vi "Write FFT Window.vi"(8 "error in (no error)":errorcluster, 10 "FFT Window":dbl, 11 "MOCKBEAR in":refnum<class "MOCKBEAR.lvclass">) -> (0 "error out":errorcluster, 3 "MOCKBEAR out":refnum<class "MOCKBEAR.lvclass">)   [LabVIEW 2021, in "MOCKBEAR.lvclass"]
uses:
  MOCKBEAR.lvclass
  MOCKBEAR.lvclass/MOCKBEAR.ctl
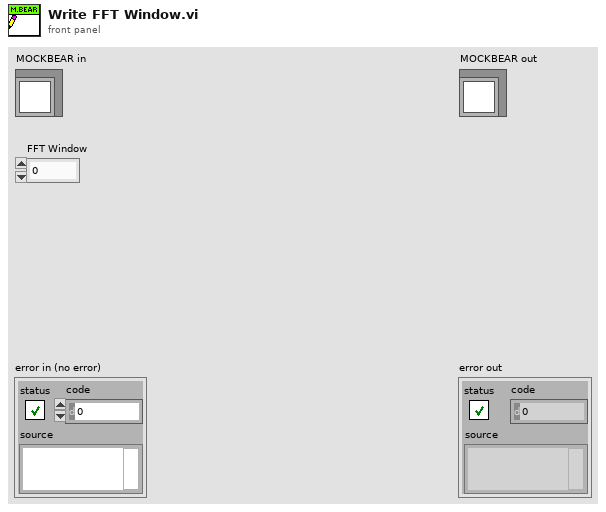
[diagram p1: front panel]
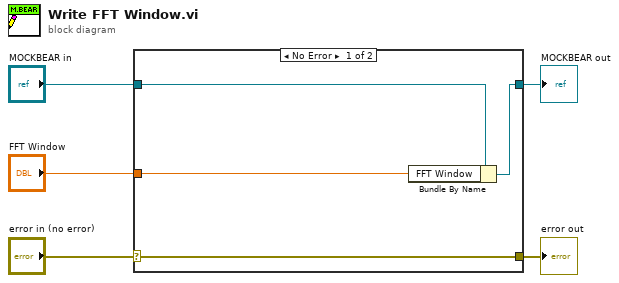
[diagram p0: block diagram]
diagram:
  n1 = case shown="No Error" "error in (no error)" {
    selector: "error in (no error)" -> [w9 w10]
    tunnel: [w9 w10] -> w4
    tunnel: [w7 w11] -> w2
    tunnel: "MOCKBEAR in" -> [w8 w11]
    tunnel: "FFT Window" -> [w6 _]
    frame No Error {
      n2 = Bundle By Name(cluster=w8, "FFT Window"=w6) -> (w7:refnum<class "MOCKBEAR.lvclass">)
    }
    frame Error {
    }
  }
  "error out" <- w4
  "MOCKBEAR out" <- w2
